vi "Create Response.vi"(8 "error in (no error)":errorcluster, 9 "result":variant, 11 "JSON-RPC in":refnum<class "JSON-RPC.lvclass">) -> (0 "error out":errorcluster, 2 "Response":string, 3 "JSON-RPC out":refnum<class "JSON-RPC.lvclass">)   [LabVIEW 2019, in "JSON-RPC.lvclass"]
uses:
  JSON-RPC.lvclass
  JSON-RPC.lvclass/JSON-RPC.ctl
  Response/Response.lvclass
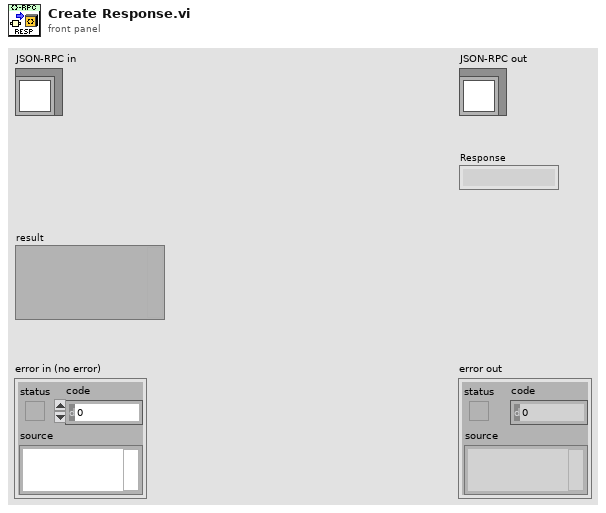
[diagram p1: front panel]
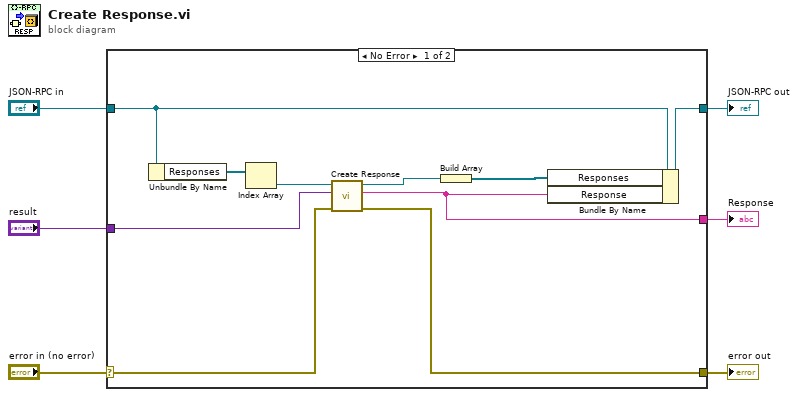
[diagram p0: block diagram]
diagram:
  n1 = case shown="No Error" "error in (no error)" {
    selector: "error in (no error)" -> [w8 w18]
    tunnel: [w13 w18] -> w5
    tunnel: [w16 w17] -> w3
    tunnel: "JSON-RPC in" -> [w12 w17]
    tunnel: "result" -> [w7 _]
    tunnel: [w15 _] -> w1
    frame No Error {
      n2 = Unbundle By Name(w12) -> ("Responses"=w11:refnum<class "Response.lvclass">[])
      n3 = Index Array(array=w11) -> (element=w10:refnum<class "Response.lvclass">)  [unwired: 1 in]
      n4 = call "Create Response.vi"("error in (no error)"=w8, "result"=w7, "Response"=w10) -> ("error out"=w13:errorcluster, "JSON Response"=w15:string, "Response out"=w14:refnum<class "Response.lvclass">)  [unwired: 6 in]
      n5 = Build Array(w14) -> (w9:refnum<class "Response.lvclass">[])
      n6 = Bundle By Name(cluster=w12, "Responses"=w9, "Response"=w15) -> (w16:refnum<class "JSON-RPC.lvclass">)
    }
    frame Error {
    }
  }
  "error out" <- w5
  "JSON-RPC out" <- w3
  "Response" <- w1
